vi "Trim_Spectra.vi"(1 "WL_UpperIndex":i32, 2 "WL_LowerIndex":i32, 3 "Image":dbl[][][](array[numeric])) -> (0 "ImageCut":dbl[][][](array[numeric]))   [LabVIEW 2020]
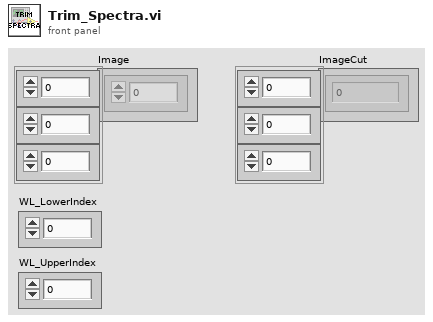
[diagram p1: front panel]
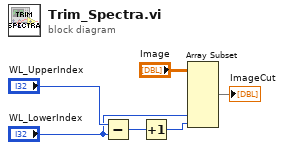
[diagram p0: block diagram]
diagram:
  n1 = Subtract(x="WL_UpperIndex", y="WL_LowerIndex") -> (x-y=w3:i32)
  n2 = Increment(x=w3) -> (x+1=w2:i32)
  n3 = Array Subset(array="Image", index (dim 2)="WL_LowerIndex", length (dim 2)=w2) -> (→"ImageCut":dbl[][][])  [unwired: 4 in]
